vi "LabVIEW Test.vi"() -> ()   [LabVIEW 2013]
uses:
  <vilib>/addons/Automotive Diagnostic Command Set/NI_Automotive Diagnostic Command Set.lvlib
  <vilib>/xnet/xnet.llb/XNET Read (Frame CAN).vi
  <vilib>/xnet/xnet.llb/XNET Frame Type CAN.ctl
  <vilib>/xnet/xnet.llb/XNET Frame CAN.ctl
  Diagnostics Add-on Custom Device.lvlib
  <vilib>/Automotive Diagnostic Command Set/Diagnostic Transport.llb/Property ID.ctl
  <vilib>/xnet/xnet.llb/XNET Database Close (Database).vi
  GMLAN/GMLAN_ReadDataByPacketIdentifier_SubFunctions.ctl
  <vilib>/xnet/xnet.llb/XNET Create Session (Frame Input Queued).vi
  <vilib>/Automotive Diagnostic Command Set/Diagnostic Transport.llb/Transport Protocol Selector.ctl
  <vilib>/Automotive Diagnostic Command Set/Diagnostic Protocols.llb/DTC Descriptor.ctl
  Program Files/National Instruments/LabVIEW 2011/examples/nixnet/examples.llb/NI-XNET Example Control - Signal.ctl
  DPID Configuration.ctl
  Shared Code/Diagnostics_DPID Periodic Rate.ctl
panel:
  out "payload":u8[](array[numeric])
  in  "Tab Control":T1(tab)
  in  "HW select":u16(ring) items=["NI-XNET", "NI-CAN"]
  in  "Transport Protocol":T2
  in  "Diagnostic Protocol":enum16{"KWP", "GMLAN"}(ring)=enum."GMLAN"
  in  "CAN Interface":string(combo)="CAN1"
  in  "Baudrate":u32=500000
  in  "Receive Address Extension":u8
  in  "Transmit Address Extension":u8
  in  "Receive ID":u32=2024 format="%.0x"
  in  "Transmit ID":u32=2016 format="%.0x"
  in  "UUDT Receive ID":u32=1512 format="%.0x"
  in  "Setup DPIDs":bool
  in  "DPIDs":T3[](array[typedef])=[{"Speed"=enum."Slow", "ID"=247, "PIDs"=[{"ID"=12, "Signals"=[{"Signal name"="EngineSpeed", "Scaling Factor"=0.25, "Scaling Offset"=0.0, "Maximum Value"=16383.75, "Minimum Value"=0.0, "Default Value"=0.0, "Unit"="V", "Start Bit"=0, "Number of Bits"=8, "Data Type"=1, "Byte Order"=0, "Comment"=""}], "Name"="EngineSpeed"}]}] {"PIDs"."Signals"."Byte Order" items=["Little Endian", "Big Endian"]; "PIDs"."Signals"."Data Type" items=["Signed", "Unsigned", "IEEE Float"]; "PIDs"."ID" format="%.0x"; "ID" format="%.0x"}
  in  "DTC descriptor":T6={"DTC Byte Length"=2, "Status Byte Length"=1, "Add Data Byte Length"=1, "Byte Order"=enum."Motorola"}
  out "data":T7[](array[typedef]) {"payload" format="%x"; "timestamp" format="%<%.7X\n%x>T"; "type" items=["CAN Data"=0, "CAN Remote"=1, "CAN Bus Error"=2, "Delay"=224, "Log Trigger"=225, "Start Trigger"=226]; "identifier" format="%x"}
  in  "DID ID":u8 format="%.0x"
  out "DID Data":u8[](array[numeric])
  in  "DID":bool
  out "PID Data":u8[](array[numeric])
  in  "PID ID":u16 format="%.0x"
  in  "Read PIDs":bool
  in  "Stop DPIDs":bool
  in  "Start DPIDs":bool
  out "DPID Setup":T3 {"PIDs"."Signals"."Byte Order" items=["Little Endian", "Big Endian"]; "PIDs"."Signals"."Data Type" items=["Signed", "Unsigned", "IEEE Float"]; "PIDs"."ID" format="%.0x"; "ID" format="%.0x"}
  out "timestamp":timestamp
  out "DTCs":T9(array[cluster]) {"Add Data" format="%.0x"; "Status" format="%.0x"; "DTC" format="%.0x"}
  in  "Read DTCs":bool
  in  "DTC Reset":bool
  out "EndofDTCReport":bool
  out "DTCCountRecord":u16
  in  "status mask":u8=1 format="%.0x"
  out "error IO":errorcluster
  out "Success?":bool
  in  "stop":bool
  out "stopped?":bool=TRUE
  # "$90 - VehicleIdentificationNumber (VIN)\n$92\t- System Supplier ID\n$97\t- SystemNameOrEngineType"
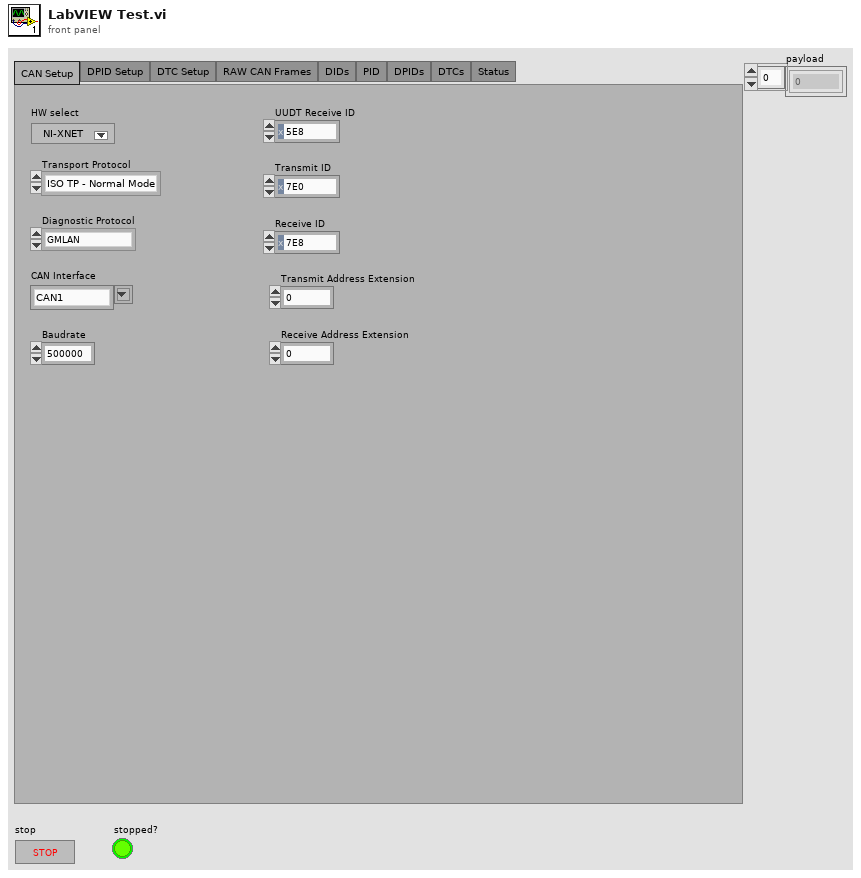
[diagram p1: front panel]
types:
  T1 = enum32{"CAN Setup", "DPID Setup", "DTC Setup", "RAW CAN Frames", "DIDs", "PID", "DPIDs", "DTCs", "Status"}
  T2 = typedef "NI_Automotive Diagnostic Command Set.lvlib/Transport Protocol Selector.ctl" = enum16{"ISO TP - Normal Mode", "ISO TP - Mixed Mode", "VW TP 2.0", "Diagnostics on IP", "ISO TP LIN"}
  T3 = typedef "DPID Configuration.ctl" = cluster{"Speed":T4, "ID":u8, "PIDs":cluster{"ID":u16, "Signals":T5[], "Name":string}[]}
  T4 = typedef "Diagnostics Add-on Custom Device.lvlib/Diagnostics_DPID Periodic Rate.ctl" = enum16{"Slow", "Medium", "Fast"}
  T5 = typedef "NI-XNET Example Control - Signal.ctl" = cluster{"Signal name":string, "Scaling Factor":dbl, "Scaling Offset":dbl, "Maximum Value":dbl, "Minimum Value":dbl, "Default Value":dbl, "Unit":string, "Start Bit":u32, "Number of Bits":u32, "Data Type":u32, "Byte Order":u32, "Comment":string}
  T6 = typedef "DTC Descriptor.ctl" = cluster{"DTC Byte Length":i32, "Status Byte Length":i32, "Add Data Byte Length":i32, "Byte Order":enum16{"Motorola", "Intel"}}
  T7 = typedef "XNET Frame CAN.ctl" = cluster{"timestamp":timestamp, "payload":u8[], "identifier":u32, "type":T8, "extended?":bool, "echo?":bool}
  T8 = typedef "XNET Frame Type CAN.ctl" = u8
  T9 = cluster{"DTC":u32, "Status":u32, "Add Data":u32}[]
  T10 = typedef "NI_Automotive Diagnostic Command Set.lvlib/Property ID.ctl" = enum16{"Timeout Diag Command", "Timeout FC (Bs)", "Timeout CF (Cr)", "Receive Block Size (BS)", "Wait Time CF (STmin)", "Max Wait Frames (N_WFTmax)", "Wait Frames to Send (N_WAIT)", "Time between Waits (T_W)", "Fill CAN Frames", "Fill Byte", "Invalid Response as Error", "Max RspPending Count", "VWTP Command Timeout", "STmin", "P2min", "Termination"}
  T11 = typedef "NI_Automotive Diagnostic Command Set.lvlib/Diag Reference.ctl" = cluster{"Diag CAN Handle":u32, "Transport Protocol":T2, "Receive Address Extension":u8, "Transmit Address Extension":u8, "Receive CAN Id":u32, "Transmit CAN Id":u32, "Diag CAN Queue":refnum<queue>, "Log Frames ?":bool, "My TP Address":u8, "Other TP Address":u8, "T1":u16, "T2":u16, "T3":u16, "T4":u16, "Tx SN":u8, "Block Size":u8, "Rx SN":u8, "VW TP Initialized?":bool, "Tx block no":u8, "baud rate":u32, "Interface":string, "Channel Diag CAN Handle":u32, "UDP Connection ID":refnum<k16>, "TCP Connection ID":refnum<k5>, "Target IP Addr":u32, "Source Address":u16, "Target Address":u16, "Send Header NACK?":bool, "DLL Handle":u32, "NAD":u8, "Time Stamp read first":dbl, "Time Stamp read last":dbl, "Time Stamp write first":dbl, "Time Stamp write last":dbl}
  T12 = enum8{"Idle", "Read DID", "Read DTCs", "Reset DTCs", "Setup DPIDs", "Start DPIDs", "Stop DPIDs", "Read PIDs", "DisableCommunication", "Stop"}
  T13 = typedef "GMLAN_ReadDataByPacketIdentifier_SubFunctions.ctl" = enum8{"stopSending", "sendOneResponse", "scheduleAtSlowRate", "scheduleAtMediumRate", "scheduleAtFastRate"}
  T14 = typedef "NI_Automotive Diagnostic Command Set.lvlib/Diag Reference.ctl" = cluster{"Diag CAN Handle":u32, "Transport Protocol":T15, "Receive Address Extension":u8, "Transmit Address Extension":u8, "Receive CAN Id":u32, "Transmit CAN Id":u32, "Diag CAN Queue":refnum<queue>, "Log Frames ?":bool, "My TP Address":u8, "Other TP Address":u8, "T1":u16, "T2":u16, "T3":u16, "T4":u16, "Tx SN":u8, "Block Size":u8, "Rx SN":u8, "VW TP Initialized?":bool, "Tx block no":u8, "baud rate":u32, "CAN interface":string, "Channel Diag CAN Handle":u32, "UDP Connection ID":refnum<k16>, "TCP Connection ID":refnum<k5>, "Target IP Addr":u32, "Source Address":u16, "Target Address":u16, "Send Header NACK?":bool}
  T15 = typedef "NI_Automotive Diagnostic Command Set.lvlib/Transport Protocol Selector.ctl" = enum16{"ISO TP - Normal Mode", "ISO TP - Mixed Mode", "VW TP 2.0", "Diagnostics on IP"}
  T16 = typedef "Diagnostic Trouble Code.ctl" = cluster{"DTC":u32, "Status":u32, "Add Data":u32}
  T17 = cluster{"ID":u16, "Signals":T5[], "Name":string}[]
  T18 = typedef "Diagnostics Add-on Custom Device.lvlib/Diagnostics_Main_Filtered DPID IDs.ctl" = cluster{"Slow":u8[], "Medium":u8[], "Fast":u8[]}
  T19 = typedef "NI_Automotive Diagnostic Command Set.lvlib/Diag CAN Frame Log.ctl" = cluster{"Timestamp":dbl, "ArbitrationId":u32, "IsRemote":u8, "DataLength":u8, "Data":u8[]}
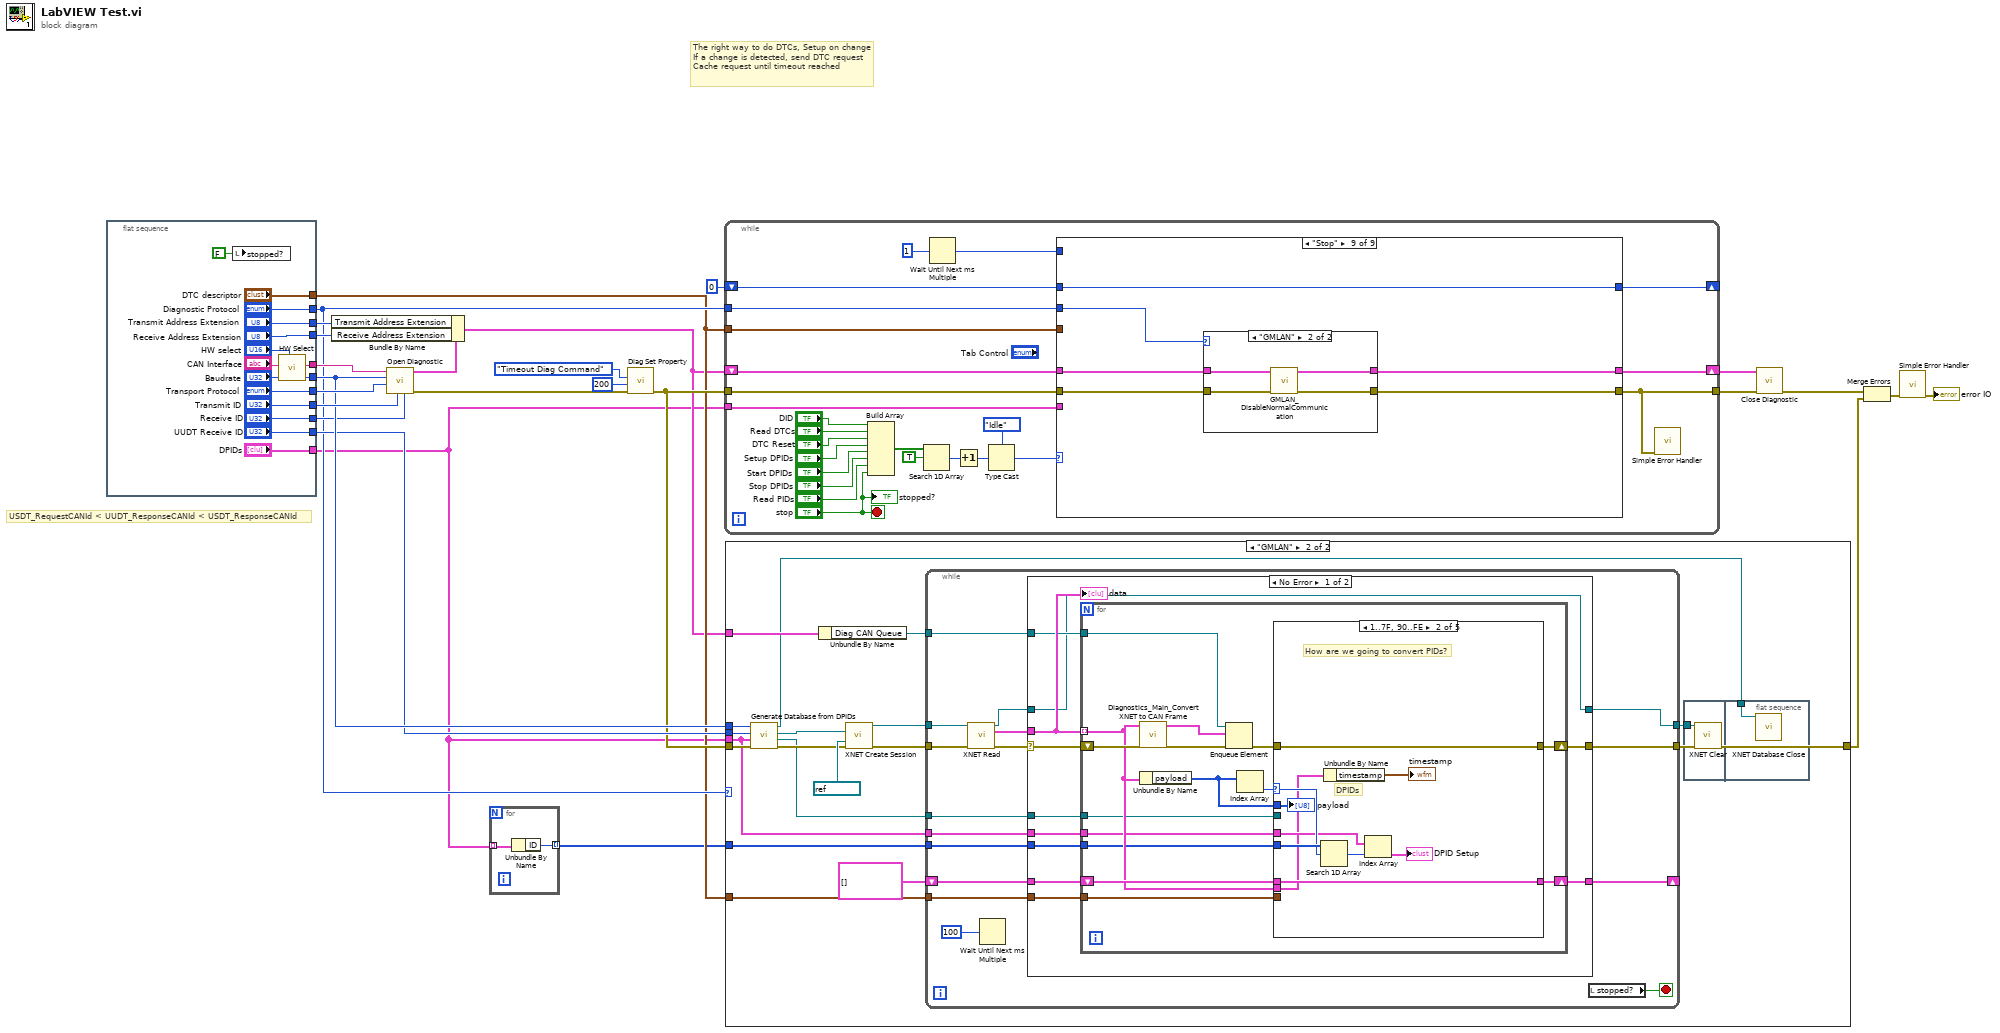
[diagram p0: block diagram]
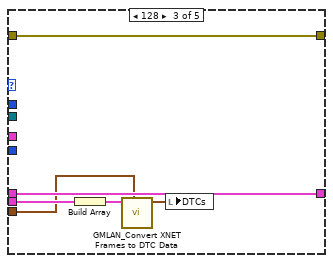
[diagram p4: hidden frame]
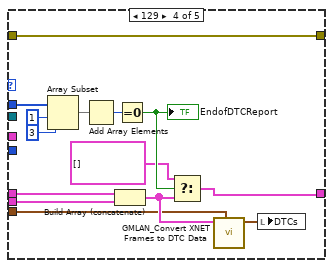
[diagram p5: hidden frame]
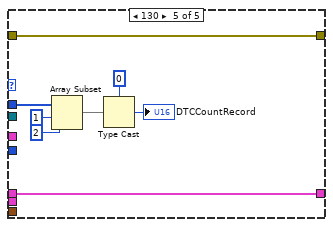
[diagram p6: hidden frame]
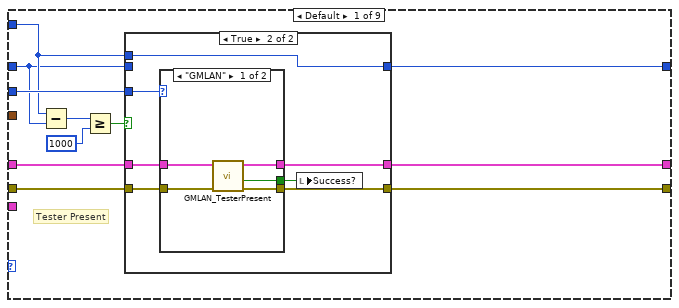
[diagram p8: hidden frame]
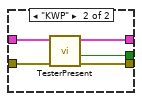
[diagram p10: hidden frame]
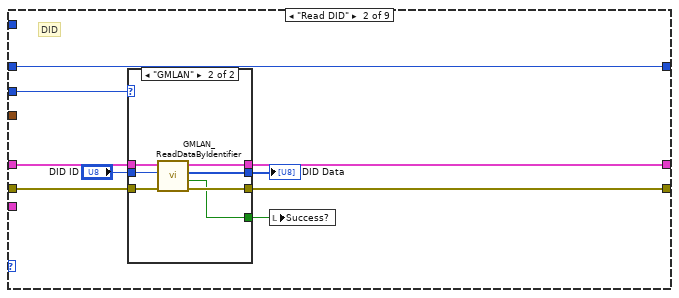
[diagram p11: hidden frame]
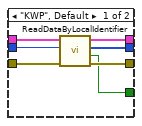
[diagram p12: hidden frame]
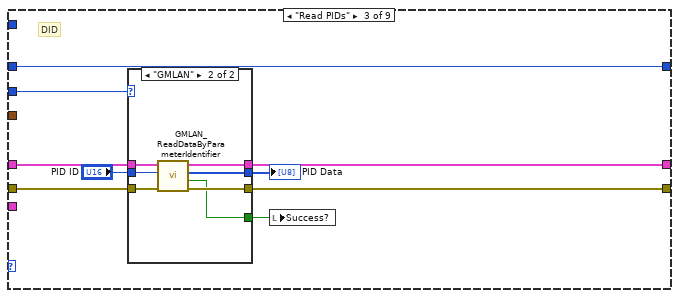
[diagram p13: hidden frame]
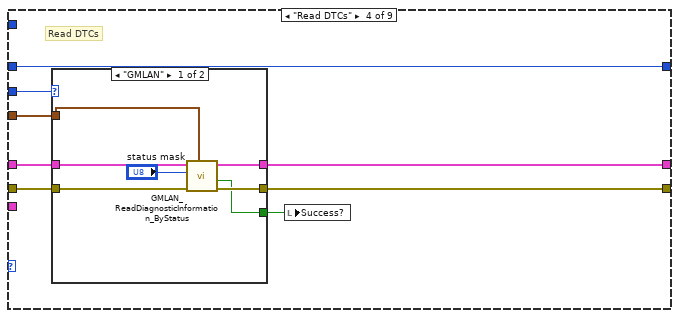
[diagram p15: hidden frame]
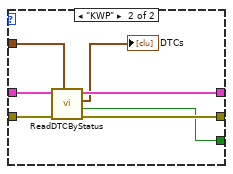
[diagram p16: hidden frame]
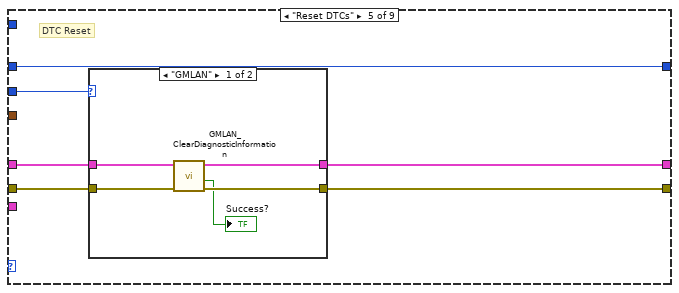
[diagram p17: hidden frame]
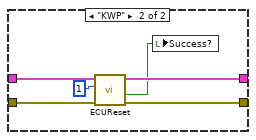
[diagram p18: hidden frame]
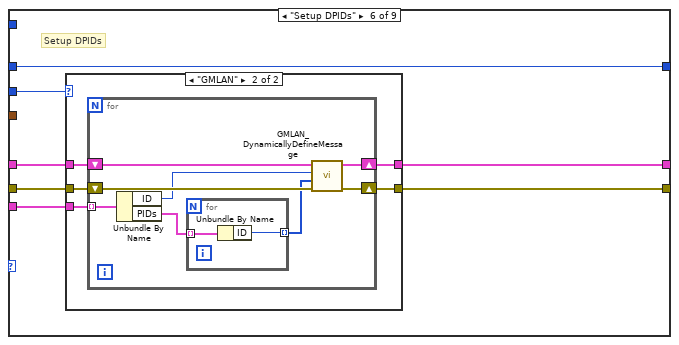
[diagram p19: hidden frame]
diagram:
  # "The right way to do DTCs, Setup on change\nIf a change is detected, send DTC request\nCache request until timeout reached"
  # "USDT_RequestCANId < UUDT_ResponseCANId < USDT_ResponseCANId"
  n1 = flat-sequence {
    tunnel: ["Transmit Address Extension"] -> w25
    tunnel: ["Receive Address Extension"] -> w24
    tunnel: [w37] -> w21
    tunnel: ["Baudrate"] -> w17
    tunnel: ["Transport Protocol"] -> w19
    tunnel: ["Transmit ID"] -> w18
    tunnel: ["Receive ID"] -> w15
    tunnel: ["Diagnostic Protocol"] -> w14
    tunnel: ["UUDT Receive ID"] -> w16
    tunnel: ["DTC descriptor"] -> w9
    tunnel: ["DPIDs"] -> w1
    frame #0 {
      n2 = local write "stopped?"(FALSE ("stopped?")) -> ()
      n3 = call "HW Select.vi"("HW select"="HW select", "CAN port"="CAN Interface") -> ("CAN port out"=w37:string)  [unwired: 9 out]
    }
  }
  n4 = call <vilib>:"Open Diagnostic.vi"("Receive ID"=w15, "Transmit ID"=w18, "Transport Protocol"=w19, "Baud Rate"=w17, "CAN Interface"=w21) -> ("error out"=w13:errorcluster, "diag ref out"=w20:T11)  [unwired: 1 in, 4 out]
  n5 = Bundle By Name(cluster=w20, "Transmit Address Extension"=w25, "Receive Address Extension"=w24) -> (w8:T11)
  n6 = for {
    tunnel: w1 -> [w41] mode=indexing
    tunnel: [w40] -> w7 mode=indexing
    n7 = Unbundle By Name(w41) -> ("ID"=w40:u8)
  }
  n8 = call <vilib>:"Diag Set Property.vi"("error in (no error)"=w13, "property value"=u32 200, "property ID"=Property_ID."Timeout Diag Command") -> ("error out"=w12:errorcluster)  [unwired: 7 in, 1 out]
  n9 = while {
    tunnel: w12 -> [w65]
    tunnel: [w42] -> w22
    shift-right: [w64] -> w23
    shift-left: w8 -> [w66]
    tunnel: w14 -> [w59]
    tunnel: w9 -> [w57]
    shift-right: [w56] -> _
    shift-left: u32 0 ("millisecond timer value") -> [w54]
    tunnel: w1 -> [w50]
    stop <- "stop" stop-if-true
    n10 = Build Array("DID", "Read DTCs", "DTC Reset", "Setup DPIDs", "Start DPIDs", "Stop DPIDs", "Read PIDs", "stop") -> (w62:bool[])
    n11 = Search 1D Array(1D array=w62, element=TRUE) -> (index of element=w47:i32)  [unwired: 1 in]
    n12 = Wait Until Next ms Multiple(millisecond multiple=1) -> (millisecond timer value=w55:u32)
    n13 = Increment(x=w47) -> (x+1=w45:u8)
    n14 = Type Cast(type=T12."Idle", x=w45) -> (*(type *) &x=w44:T12)
    n15 = case shown="\"Stop\"" w44 {
      tunnel: w66 -> [w76 w105 w128 w143 w166 w181 w206 w244 w271]
      tunnel: w65 -> [w77 w104 w127 w145 w165 w183 w208 w246 w272]
      tunnel: [w74 w103 w126 w142 w164 w180 w205 w243 w269] -> w64
      tunnel: [w75 w102 w125 w144 w163 w182 w207 w245 w270] -> w42
      tunnel: w59 -> [w73 w106 w129 w146 w162 w178 w202 w240 w267]
      tunnel: w57 -> [_ _ _ w140 _ _ _ _ _]
      tunnel: w55 -> [w71 _ _ _ _ _ _ _ _]
      tunnel: [w72 w98 w121 w139 w161 w184 w204 w242 w268] -> w56
      tunnel: w54 -> [w67 w98 w121 w139 w161 w184 w204 w242 w268]
      tunnel: w50 -> [_ _ _ _ _ w179 w203 w241 _]
      frame Default {
        # "Tester Present"
        n16 = Subtract(x=w71, y=w67) -> (x-y=w70:u32)
        n17 = Greater Or Equal?(x=w70, y=u32 1000) -> (x >= y?=w68:bool)
        n18 = case shown="True" w68 {
          tunnel: w77 -> [w79 w87]
          tunnel: w76 -> [w80 w86]
          tunnel: [w79 w85] -> w75
          tunnel: [w80 w84] -> w74
          tunnel: w73 -> [_ w82]
          tunnel: w71 -> [_ w81]
          tunnel: [w78 w81] -> w72
          tunnel: w67 -> [w78 _]
          frame False {
          }
          frame True {
            n19 = case shown="\"GMLAN\"" w82 {
              tunnel: w87 -> [w92 w97]
              tunnel: w86 -> [w91 w96]
              tunnel: [w89 w95] -> w85
              tunnel: [w90 w94] -> w84
              tunnel: [w88 w93] -> w83
              frame "GMLAN" {
                n20 = call "GMLAN_TesterPresent.vi"("error in (no error)"=w92, "diag ref in"=w91) -> ("error out"=w89:errorcluster, "success?"=w88:bool, "diag ref out"=w90:T14)  [unwired: 7 in]
              }
              frame "KWP" {
                n21 = call <vilib>:"TesterPresent.vi"("error in (no error)"=w97, "diag ref in"=w96) -> ("error out"=w95:errorcluster, "success?"=w93:bool, "diag ref out"=w94:T11)  [unwired: 3 in, 4 out]
              }
            }
            n22 = local write "Success?"(w83) -> ()
          }
        }
      }
      frame "Read DID" {
        # "DID"
        n23 = case shown="\"GMLAN\"" w106 {
          tunnel: w105 -> [w113 w120]
          tunnel: w104 -> [w112 w119]
          tunnel: [w110 w118] -> w103
          tunnel: [w111 w117] -> w102
          tunnel: [w109 w115] -> w99
          tunnel: [w108 w116] -> w101
          tunnel: "DID ID" -> [w107 w114]
          frame "KWP", Default {
            n24 = call <vilib>:"ReadDataByLocalIdentifier.vi"("error in (no error)"=w112, "local ID"=w107, "diag ref in"=w113) -> ("error out"=w111:errorcluster, "success?"=w108:bool, "data out"=w109:u8[], "diag ref out"=w110:T11)  [unwired: 5 in]
          }
          frame "GMLAN" {
            n25 = call "GMLAN_ReadDataByIdentifier.vi"("error in (no error)"=w119, "Data ID (DID)"=w114, "diag ref in"=w120) -> ("error out"=w117:errorcluster, "success?"=w116:bool, "data out"=w115:u8[], "diag ref out"=w118:T14)  [unwired: 5 in]
          }
        }
        "DID Data" <- w99
        n26 = local write "Success?"(w101) -> ()
      }
      frame "Read PIDs" {
        # "DID"
        n27 = case shown="\"GMLAN\"" w129 {
          tunnel: w128 -> [w130 w138]
          tunnel: w127 -> [w131 w137]
          tunnel: [w130 w136] -> w126
          tunnel: [w131 w135] -> w125
          tunnel: [_ w133] -> w122
          tunnel: [_ w134] -> w124
          tunnel: "PID ID" -> [_ w132]
          frame "KWP", Default {
          }
          frame "GMLAN" {
            n28 = call "GMLAN_ReadDataByParameterIdentifier.vi"("error in (no error)"=w137, "Parameter ID (PID)"=w132, "diag ref in"=w138) -> ("error out"=w135:errorcluster, "success?"=w134:bool, "data out"=w133:u8[], "diag ref out"=w136:T14)  [unwired: 5 in]
          }
        }
        "PID Data" <- w122
        n29 = local write "Success?"(w124) -> ()
      }
      frame "Read DTCs" {
        # "Read DTCs"
        n30 = case shown="\"GMLAN\"" w146 {
          tunnel: w145 -> [w153 w160]
          tunnel: [w152 w159] -> w144
          tunnel: w143 -> [w150 w158]
          tunnel: [w151 w157] -> w142
          tunnel: [w149 w156] -> w141
          tunnel: w140 -> [w148 w155]
          frame "GMLAN" {
            n31 = call "GMLAN_ReadDiagnosticInformation_ByStatus.vi"(7:w148, "error in (no error)"=w153, "status mask"="status mask", "diag ref in"=w150) -> ("error out"=w152:errorcluster, "success?"=w149:bool, "diag ref out"=w151:T14)  [unwired: 4 in, 1 out]
          }
          frame "KWP" {
            n32 = call <vilib>:"ReadDTCByStatus.vi"("DTC descriptor"=w155, "error in (no error)"=w160, "diag ref in"=w158) -> ("error out"=w159:errorcluster, "success?"=w156:bool, "DTCs"=→"DTCs":T16[], "diag ref out"=w157:T11)  [unwired: 5 in]
          }
        }
        n33 = local write "Success?"(w141) -> ()
      }
      frame "Reset DTCs" {
        # "DTC Reset"
        n34 = case shown="\"GMLAN\"" w162 {
          tunnel: w166 -> [w169 w177]
          tunnel: w165 -> [w171 w176]
          tunnel: [w168 w175] -> w164
          tunnel: [w170 w174] -> w163
          frame "GMLAN" {
            n35 = call "GMLAN_ClearDiagnosticInformation.vi"("error in (no error)"=w171, "diag ref in"=w169) -> ("error out"=w170:errorcluster, "success?"=→"Success?":bool, "diag ref out"=w168:T14)  [unwired: 7 in]
          }
          frame "KWP" {
            n36 = call <vilib>:"ECUReset.vi"("error in (no error)"=w176, "mode"=u8 1 ("Mode"), "diag ref in"=w177) -> ("error out"=w174:errorcluster, "success?"=w173:bool, "diag ref out"=w175:T11)  [unwired: 2 in, 4 out]
            n37 = local write "Success?"(w173) -> ()
          }
        }
      }
      frame "Setup DPIDs" {
        # "Setup DPIDs"
        n38 = case shown="\"GMLAN\"" w178 {
          tunnel: w183 -> [w185 w191]
          tunnel: [w185 w190] -> w182
          tunnel: w181 -> [w186 w189]
          tunnel: [w186 w188] -> w180
          tunnel: w179 -> [_ w187]
          frame "KWP", Default {
          }
          frame "GMLAN" {
            n39 = for {
              shift-right: [w198] -> w190
              shift-left: w191 -> [w199]
              shift-right: [w196] -> w188
              shift-left: w189 -> [w197]
              tunnel: w187 -> [w195] mode=indexing
              n40 = Unbundle By Name(w195) -> ("ID"=w193:u8, "PIDs"=w194:T17)
              n41 = for {
                tunnel: w194 -> [w201] mode=indexing
                tunnel: [w200] -> w192 mode=indexing
                n42 = Unbundle By Name(w201) -> ("ID"=w200:u16)
              }
              n43 = call "GMLAN_DynamicallyDefineMessage.vi"("error in (no error)"=w199, "PID List"=w192, "DPID ID"=w193, "diag ref in"=w197) -> ("error out"=w198:errorcluster, "diag ref out"=w196:T14)  [unwired: 5 in, 1 out]
            }
          }
        }
      }
      frame "Start DPIDs" {
        # "Start DPIDs"
        n44 = case shown="\"GMLAN\"" w202 {
          tunnel: w208 -> [w209 w217]
          tunnel: [w209 w216] -> w207
          tunnel: w206 -> [w210 w215]
          tunnel: [w210 w214] -> w205
          tunnel: w203 -> [_ w213]
          frame "KWP", Default {
          }
          frame "GMLAN" {
            w211 = T13[] [enum."scheduleAtSlowRate", enum."scheduleAtMediumRate", enum."scheduleAtFastRate"] items=["stopSending", "sendOneResponse", "scheduleAtSlowRate", "scheduleAtMediumRate", "scheduleAtFastRate"]
            n45 = call "Diagnostics_Sort DPID IDs by Speed.vi"("DPIDs"=w213) -> ("Filtered DPIDs IDs"=w212:T18)  [unwired: 10 in]
            n46 = for {
              tunnel: w212 -> [w221]
              shift-right: [w224] -> w216
              shift-left: w217 -> [w225]
              shift-right: [w222] -> w214
              shift-left: w215 -> [w223]
              tunnel: w211 -> [w218] mode=indexing
              n47 = case shown="\"scheduleAtMediumRate\"" w218 {
                tunnel: w221 -> [w235 w237 _ w239]
                tunnel: [w234 w236 _ w238] -> w220
                frame "scheduleAtMediumRate" {
                  n48 = Unbundle By Name(w235) -> ("Medium"=w234:u8[])
                }
                frame "scheduleAtFastRate" {
                  n49 = Unbundle By Name(w237) -> ("Fast"=w236:u8[])
                }
                frame Default {
                }
                frame "scheduleAtSlowRate" {
                  n50 = Unbundle By Name(w239) -> ("Slow"=w238:u8[])
                }
              }
              n51 = Empty Array?(array=w220) -> (empty?=w219:bool)
              n52 = case shown="False" w219 {
                tunnel: w225 -> [w231 w232]
                tunnel: [w230 w232] -> w224
                tunnel: w223 -> [w229 w233]
                tunnel: [w228 w233] -> w222
                tunnel: w218 -> [w227 _]
                tunnel: w220 -> [w226 _]
                frame False {
                  n53 = call "GMLAN_ReadDataByPacketIdentifier.vi"("error in (no error)"=w231, "DPIDs"=w226, "Sub Function"=w227, "diag ref in"=w229) -> ("error out"=w230:errorcluster, "diag ref out"=w228:T14)  [unwired: 4 in, 2 out]
                }
                frame True {
                }
              }
            }
          }
        }
      }
      frame "Stop DPIDs" {
        # "Start DPIDs"
        n54 = case shown="\"GMLAN\"" w240 {
          tunnel: w246 -> [w247 w256]
          tunnel: [w247 w255] -> w245
          tunnel: w244 -> [w248 w254]
          tunnel: [w248 w253] -> w243
          tunnel: w241 -> [_ w252]
          frame "KWP", Default {
          }
          frame "GMLAN" {
            n55 = for {
              tunnel: w252 -> [w266] mode=indexing
              tunnel: [w265] -> w250 mode=indexing
              n56 = Unbundle By Name(w266) -> ("ID"=w265:u8)
            }
            n57 = Empty Array?(array=w250) -> (empty?=w251:bool)
            n58 = case shown="False" w251 {
              tunnel: w256 -> [w262 w263]
              tunnel: [w261 w263] -> w255
              tunnel: w254 -> [w260 w264]
              tunnel: [w259 w264] -> w253
              tunnel: GMLAN_ReadDataByPacketIdentifier_SubFunctions."stopSending" ("Sub Function") -> [w258 _]
              tunnel: w250 -> [w257 _]
              frame False {
                n59 = call "GMLAN_ReadDataByPacketIdentifier.vi"("error in (no error)"=w262, "DPIDs"=w257, "Sub Function"=w258, "diag ref in"=w260) -> ("error out"=w261:errorcluster, "diag ref out"=w259:T14)  [unwired: 4 in, 2 out]
              }
              frame True {
              }
            }
          }
        }
      }
      frame "Stop" {
        n60 = case shown="\"GMLAN\"" w267 {
          tunnel: w272 -> [w274 w278]
          tunnel: w271 -> [w273 w277]
          tunnel: [w274 w276] -> w270
          tunnel: [w273 w275] -> w269
          frame "KWP", Default {
          }
          frame "GMLAN" {
            n61 = call "GMLAN_DisableNormalCommunication.vi"("error in (no error)"=w278, "diag ref in"=w277) -> ("error out"=w276:errorcluster, "diag ref out"=w275:T14)  [unwired: 7 in, 1 out]
          }
        }
      }
    }
    n62 = call <vilib>:"Simple Error Handler.vi"("error in (no error)"=w42) -> ()  [unwired: 4 in, 5 out]
    "stopped?" <- "stop"
  }
  n63 = case shown="\"GMLAN\"" w14 {
    tunnel: w12 -> [w279 w291]
    tunnel: w17 -> [_ w290]
    tunnel: w16 -> [_ w289]
    tunnel: w8 -> [_ w294]
    tunnel: w9 -> [_ w292]
    tunnel: [w279 w282] -> w5
    tunnel: w1 -> [_ w286]
    tunnel: w7 -> [_ w285]
    frame "KWP", Default {
    }
    frame "GMLAN" {
      n64 = call "Generate Database from DPIDs.vi"("error in (no error)"=w291, "DPIDs"=w286, "UUDT Receive ID"=w289, "Baud Rate"=w290) -> ("error out"=w288:errorcluster, "Conversion Session"=w280:refnum<k21>, "frame out"=w284:refnum<k21>, "database out"=w281:refnum<k21>)  [unwired: 4 in]
      n65 = Unbundle By Name(w294) -> ("Diag CAN Queue"=w293:refnum<queue>)
      n66 = call-poly <vilib>:"XNET Create Session.vi"("frame"=w284, "interface"=refnum<k21> "CAN1", "error in (no error)"=w288) -> ("session out"=w283:refnum<k21>, "error out"=w296:errorcluster)  [unwired: 11 out]
      n67 = while {
        tunnel: w296 -> [w312]
        shift-right: [w308] -> _
        shift-left: T7[] [] ("data") -> [w309]
        tunnel: w293 -> [w307]
        tunnel: w292 -> [w306]
        tunnel: [w304] -> w282
        tunnel: w286 -> [w303]
        tunnel: w285 -> [w302]
        tunnel: w283 -> [w313]
        tunnel: [w301] -> w287
        tunnel: w280 -> [w300]
        stop <- w315 stop-if-true
        n68 = call-poly <vilib>:"XNET Read.vi"("session in"=w313, "error in (no error)"=w312) -> ("session out"=w305:refnum<k21>, "data"=w310:T7[], "error out"=w311:errorcluster)  [unwired: 10 in, 1 out]
        n69 = Wait Until Next ms Multiple(millisecond multiple=100) -> ()  [unwired: 1 out]
        n70 = case shown="No Error" w311 {
          selector: w311 -> [w323 w383]
          tunnel: w310 -> [w326 _]
          tunnel: [w322 w383] -> w304
          tunnel: w309 -> [w325 w382]
          tunnel: [w324 w382] -> w308
          tunnel: w307 -> [w321 _]
          tunnel: w306 -> [w320 _]
          tunnel: w305 -> [w317 w381]
          tunnel: w303 -> [w319 _]
          tunnel: w302 -> [w318 _]
          tunnel: [w317 w381] -> w301
          tunnel: w300 -> [w316 _]
          frame No Error {
            n71 = for {
              tunnel: w326 -> [w332] mode=indexing
              shift-right: [w338] -> w324
              shift-left: w325 -> [w339]
              shift-right: [w337] -> w322
              shift-left: w323 -> [w336]
              tunnel: w321 -> [w334]
              tunnel: w320 -> [w330]
              tunnel: w319 -> [w329]
              tunnel: w318 -> [w328]
              tunnel: w316 -> [w327]
              n72 = Unbundle By Name(w332) -> ("payload"=w331:u8[])
              n73 = call "Diagnostics_Main_Convert XNET to CAN Frame.vi"("XNET frame"=w332) -> ("CAN Frame"=w333:T19)  [unwired: 10 in]
              n74 = Enqueue Element(queue=w334, element=w333, error in (no error)=w336) -> (error out=w335:errorcluster)  [unwired: 1 in, 2 out]
              n75 = Index Array(array=w331) -> (element=w340:u8)  [unwired: 1 in]
              n76 = case shown="1..7F, 90..FE" w340 {
                selector: w340 -> [_ w350 _ _ _]
                tunnel: w331 -> [_ w343 _ w372 w376]
                tunnel: w339 -> [w342 w352 w358 w366 w380]
                tunnel: w332 -> [_ w346 w356 w365 _]
                tunnel: [w342 w352 w358 w363 w380] -> w338
                tunnel: [w341 w344 w357 w362 w379] -> w337
                tunnel: w335 -> [w341 w344 w357 w362 w379]
                tunnel: w330 -> [_ _ w354 w360 _]
                tunnel: w329 -> [_ w348 _ _ _]
                tunnel: w328 -> [_ w351 _ _ _]
                tunnel: w327 -> [_ _ _ _ _]
                frame Default {
                }
                frame 1..127, 144..254 {
                  # "How are we going to convert PIDs?"
                  # "DPIDs"
                  n77 = Search 1D Array(1D array=w351, element=w350) -> (index of element=w349:i32)  [unwired: 1 in]
                  n78 = Unbundle By Name(w346) -> ("timestamp"=→"timestamp":timestamp)
                  n79 = Index Array(array=w348, index=w349) -> (element=→"DPID Setup":T3)
                  "payload" <- w343
                }
                frame 128 {
                  n80 = Build Array(w356) -> (w355:T7[])
                  n81 = call "GMLAN_Convert XNET Frames to DTC Data.vi"("DTC descriptor"=w354, "All DTCs"=w355) -> ("DTCs"=w353:T16[])  [unwired: 9 in]
                  n82 = local write "DTCs"(w353) -> ()
                }
                frame 129 {
                  n83 = Array Subset(array=w372, index=1, length=3) -> (w369:u8[])
                  n84 = Add Array Elements(numeric array=w369) -> (sum=w368:u8)
                  n85 = Build Array (concatenate)(w366, w365) -> (w361:T7[])
                  n86 = Equal To 0?(x=w368) -> (x = 0?=w367:bool)
                  "EndofDTCReport" <- w367
                  n87 = Select(t=T7[] [] ("data"), s=w367, f=w361) -> (s? t:f=w363:T7[])
                  n88 = call "GMLAN_Convert XNET Frames to DTC Data.vi"("DTC descriptor"=w360, "All DTCs"=w361) -> ("DTCs"=w359:T16[])  [unwired: 9 in]
                  n89 = local write "DTCs"(w359) -> ()
                }
                frame 130 {
                  n90 = Array Subset(array=w376, index=1, length=2) -> (w375:u8[])
                  n91 = Type Cast(type=u16 0 ("length"), x=w375) -> (*(type *) &x=→"DTCCountRecord":u16)
                }
              }
            }
            "data" <- w326
          }
          frame Error {
          }
        }
        n92 = local read "stopped?"() -> (w315:bool)
      }
      n93 = flat-sequence {
        tunnel: w287 -> [w298]
        tunnel: w281 -> [w299]
        frame #0 {
          n94 = call <vilib>:"XNET Clear.vi"("session in"=w298) -> ()  [unwired: 14 in, 1 out]
        }
        frame #1 {
          n95 = call-poly <vilib>:"XNET Database Close.vi"("database in"=w299) -> ()  [unwired: 14 in, 1 out]
        }
      }
    }
  }
  n96 = call <vilib>:"Close Diagnostic.vi"("error in (no error)"=w22, "diag ref in"=w23) -> ("error out"=w6:errorcluster)  [unwired: 9 out]
  n97 = Merge Errors(w6, w5) -> (w4:errorcluster)
  n98 = call <vilib>:"Simple Error Handler.vi"("error in (no error)"=w4) -> ("error out"=→"error IO":errorcluster)  [unwired: 1 in, 7 out]
